vi "prependTimestamp.vi"(1 "timestamp (current)":timestamp, 7 "string in":string, 12 "time format (%H:%M)":string="%H:%M") -> (8 "string out":string="Closing program")   [LabVIEW 2015]
doc: "Prepends current timestamp to a string."
panel:
  out "use current timestamp?":bool
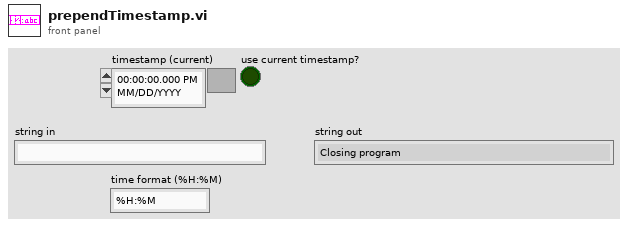
[diagram p1: front panel]
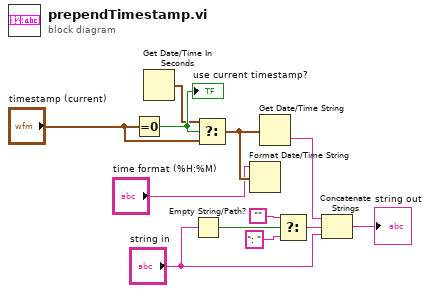
[diagram p0: block diagram]
diagram:
  n1 = Equal To 0?(x="timestamp (current)") -> (x = 0?=w5:bool)
  "use current timestamp?" <- w5
  n2 = Get Date/Time In Seconds() -> (seconds since 1Jan1904=w3:timestamp)
  n3 = Empty String/Path?(string/path="string in") -> (empty?=w9:bool)
  n4 = Select(t=w3, s=w5, f="timestamp (current)") -> (s? t:f=w2:timestamp)
  n5 = Format Date/Time String(time format string (%c)="time format (%H:%M)", seconds (now)=w2) -> ()  [unwired: 1 in, 1 out]
  n6 = Get Date/Time String(seconds (now)=w2) -> (time string=w12:string)  [unwired: 2 in, 1 out]
  n7 = Select(t="", s=w9, f=": " ("string")) -> (s? t:f=w6:string)
  n8 = Concatenate Strings(w12, w6, "string in") -> (→"string out":string)
